vi "rosbridge.vi"() -> ()   [LabVIEW 2015]
uses:
  szablon odometry_filtered_local.ctl
  Gobal for ROS.vi
  Zmienne/longitude.vi
  Zmienne/latitude.vi
  szablon odometry_filtered_local.vi
  <vilib>/Intelligent Energy/WebSockets API/WebSockets/WebSockets.lvlib
  Zmienne globalne.lvlib
panel:
  out "x-y":u32
  out "value 2":T1
  in  "szablon odometry/filtered/local":T1
  in  "ROS data IMU":T2={"topic"="", "msg"={"header"={"seq"=63049, "stamp"={"secs"=0, "nsecs"=0}, "frame_id"="imu_link"}, "orientation"={"x"=0.0, "y"=0.0, "z"=0.0, "w"=0.0}, "orientation_covariance"=[], "angular_velocity"={"x"=0.0, "y"=0.0, "z"=0.0}, "angular_velocity_covariance"=[], "linear_acceleration"={"x"=0.0, "y"=0.0, "z"=0.0}, "linear_acceleration_covariance"=[]}, "op"=""}
  out "raw frame 2":string
  in  "STOP ROS READ 2":bool
  in  "ROS data read prędkości kół":T3
  out "error out 3":errorcluster
  in  "Topic string 2":string="{ \"op\": \"subscribe\", \"topic\" : \"/odometry/filtered/local\" }"
  in  "ROSB READ 2":bool
  in  "ROS data read 3":T4
  out "ROS data read 2":T5
  out "raw frame":string
  in  "STOP ROS READ":bool
  out "value":T6
  out "ROS data read":T7
  out "error out 2":errorcluster
  in  "Topic string":string="{ \"op\": \"subscribe\", \"topic\" : \"/fix\" }"
  in  "ROSB READ":bool
  # "Topic /fix na gpsa \ntopic rio/odom na prędkości\nIMU /data"
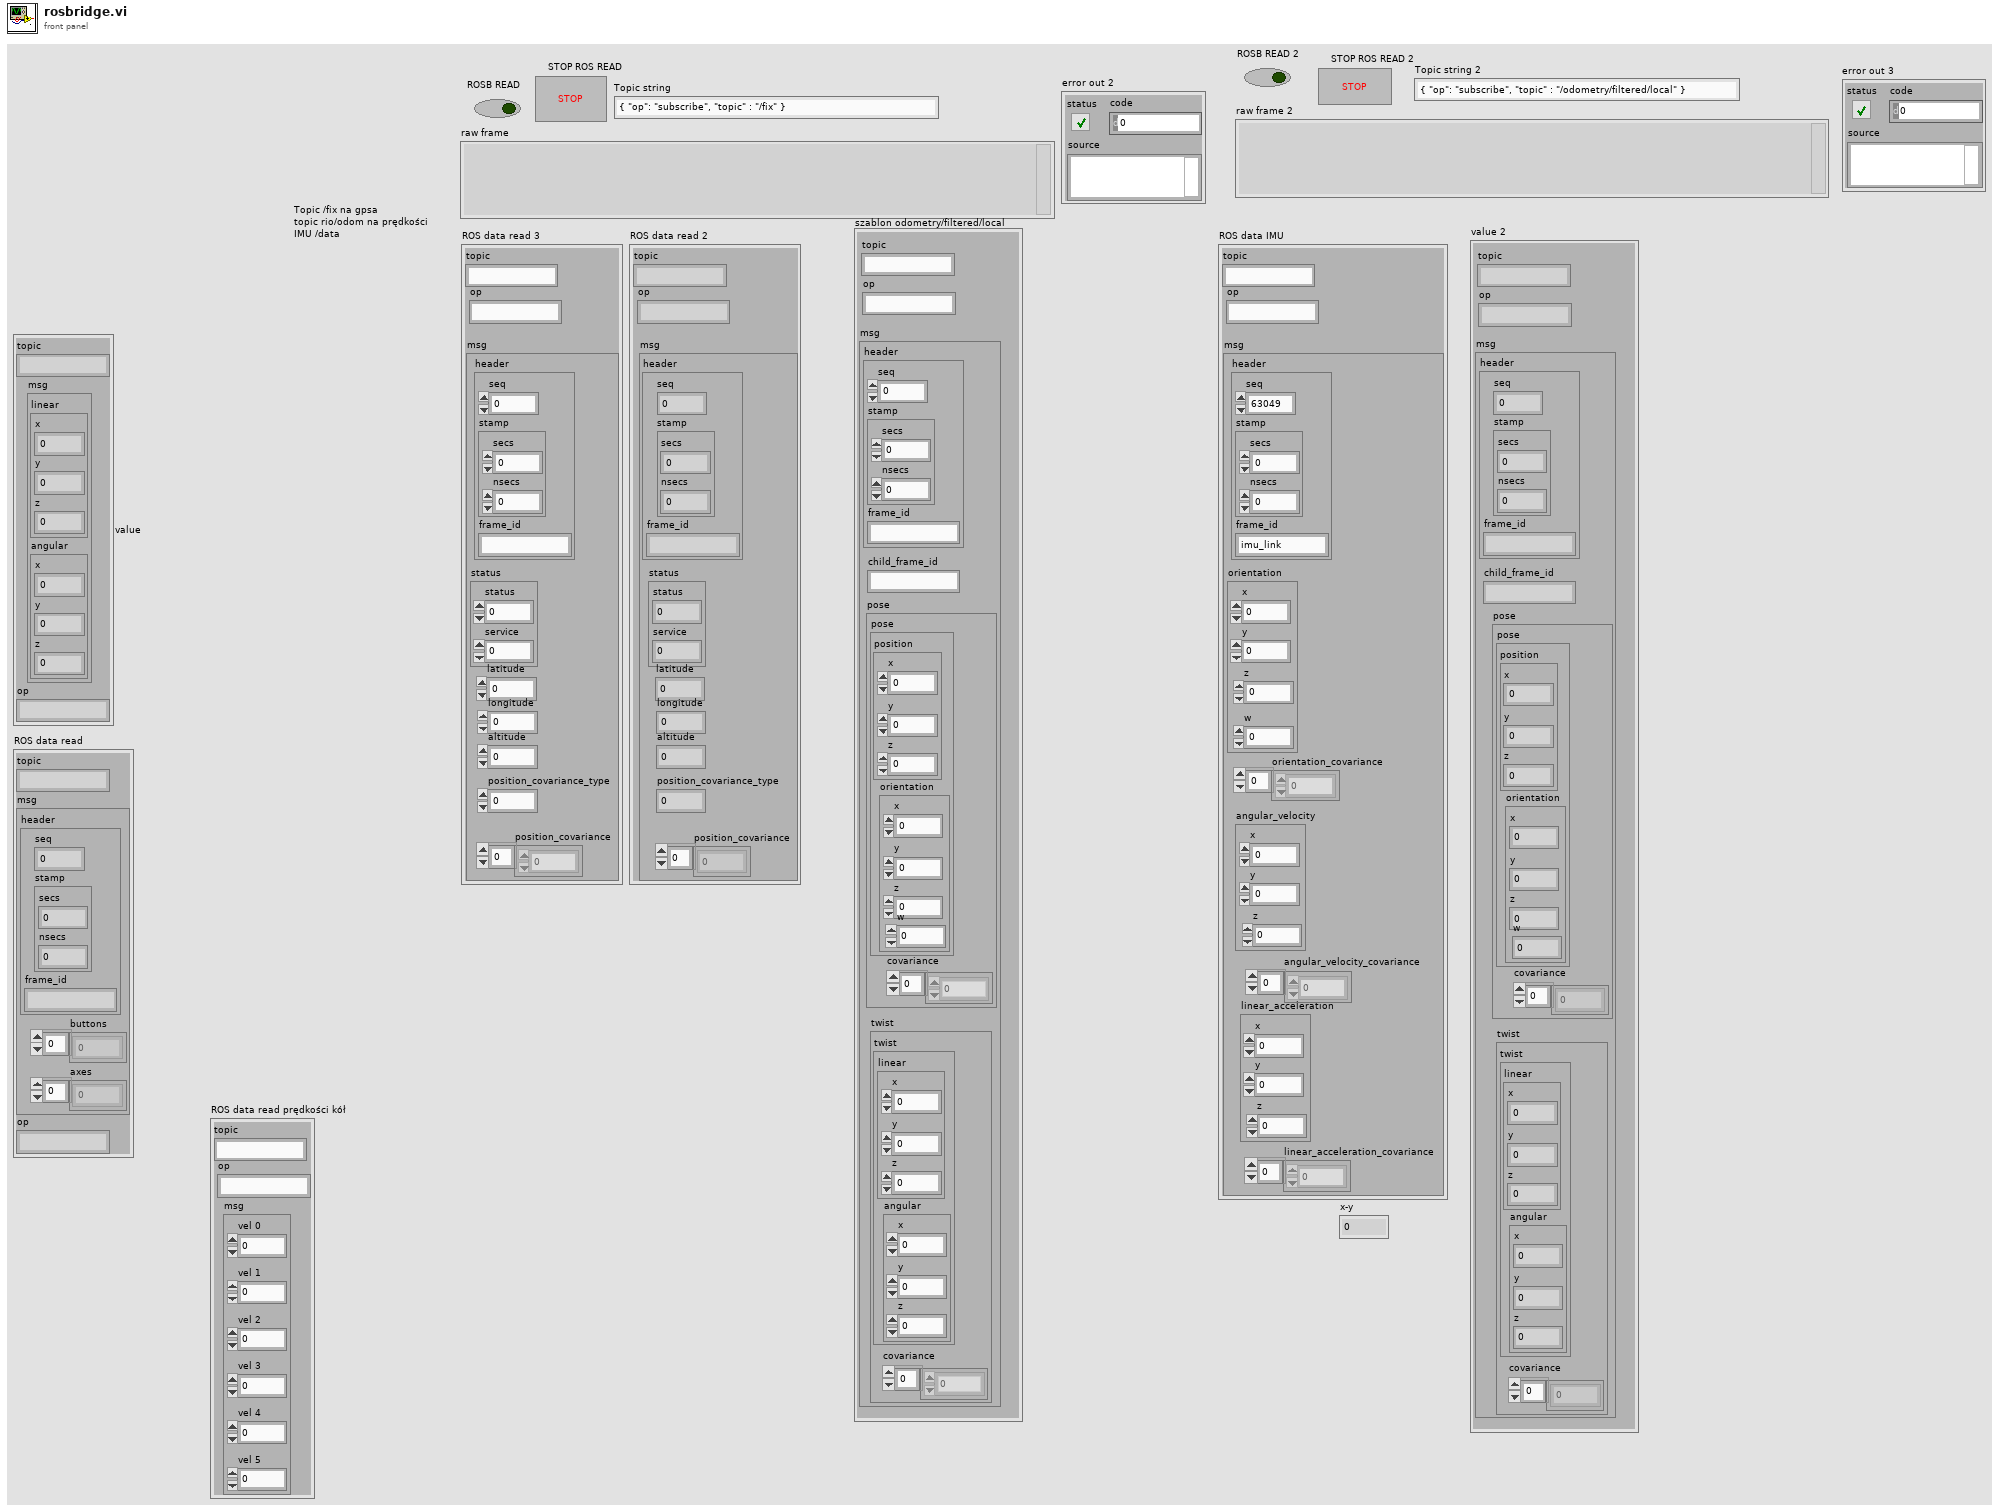
[diagram p1: front panel]
types:
  T1 = typedef "Biblioteka moduł map v3.lvlib/Zmienne globalne.lvlib/szablon odometry_filtered_local.ctl" = cluster{"topic":string, "msg":cluster{"header":cluster{"seq":u32, "stamp":cluster{"secs":u32, "nsecs":i32}, "frame_id":string}, "child_frame_id":string, "pose":cluster{"pose":cluster{"position":cluster{"y":dbl, "z":dbl, "x":dbl}, "orientation":cluster{"y":dbl, "z":dbl, "x":dbl, "w":dbl}}, "covariance":dbl[]}, "twist":cluster{"twist":cluster{"linear":cluster{"y":dbl, "z":dbl, "x":dbl}, "angular":cluster{"y":dbl, "z":dbl, "x":dbl}}, "covariance":dbl[]}}, "op":string}
  T2 = cluster{"topic":string, "msg":cluster{"header":cluster{"seq":u32, "stamp":cluster{"secs":u32, "nsecs":i32}, "frame_id":string}, "orientation":cluster{"x":dbl, "y":dbl, "z":dbl, "w":dbl}, "orientation_covariance":dbl[], "angular_velocity":cluster{"x":dbl, "y":dbl, "z":dbl}, "angular_velocity_covariance":dbl[], "linear_acceleration":cluster{"x":dbl, "y":dbl, "z":dbl}, "linear_acceleration_covariance":dbl[]}, "op":string}
  T3 = cluster{"topic":string, "msg":cluster{"vel 0":i64, "vel 1":i64, "vel 2":i64, "vel 3":i64, "vel 4":i64, "vel 5":i64}, "op":string}
  T4 = cluster{"topic":string, "msg":cluster{"header":cluster{"seq":u32, "stamp":cluster{"secs":u32, "nsecs":i32}, "frame_id":string}, "status":cluster{"status":u32, "service":i32}, "position_covariance":dbl[], "latitude":dbl, "longitude":dbl, "altitude":i32, "position_covariance_type":dbl}, "op":string}
  T5 = cluster{"topic":string, "msg":cluster{"header":cluster{"seq":u32, "stamp":cluster{"secs":u32, "nsecs":i32}, "frame_id":string}, "status":cluster{"status":u32, "service":i32}, "position_covariance":sgl[], "latitude":dbl, "longitude":dbl, "altitude":i32, "position_covariance_type":i32}, "op":string}
  T6 = cluster{"topic":string, "msg":cluster{"linear":cluster{"x":dbl, "y":dbl, "z":dbl}, "angular":cluster{"x":dbl, "y":dbl, "z":dbl}}, "op":string}
  T7 = cluster{"topic":string, "msg":cluster{"header":cluster{"seq":u32, "stamp":cluster{"secs":u32, "nsecs":i32}, "frame_id":string}, "buttons":i32[], "axes":sgl[]}, "op":string}
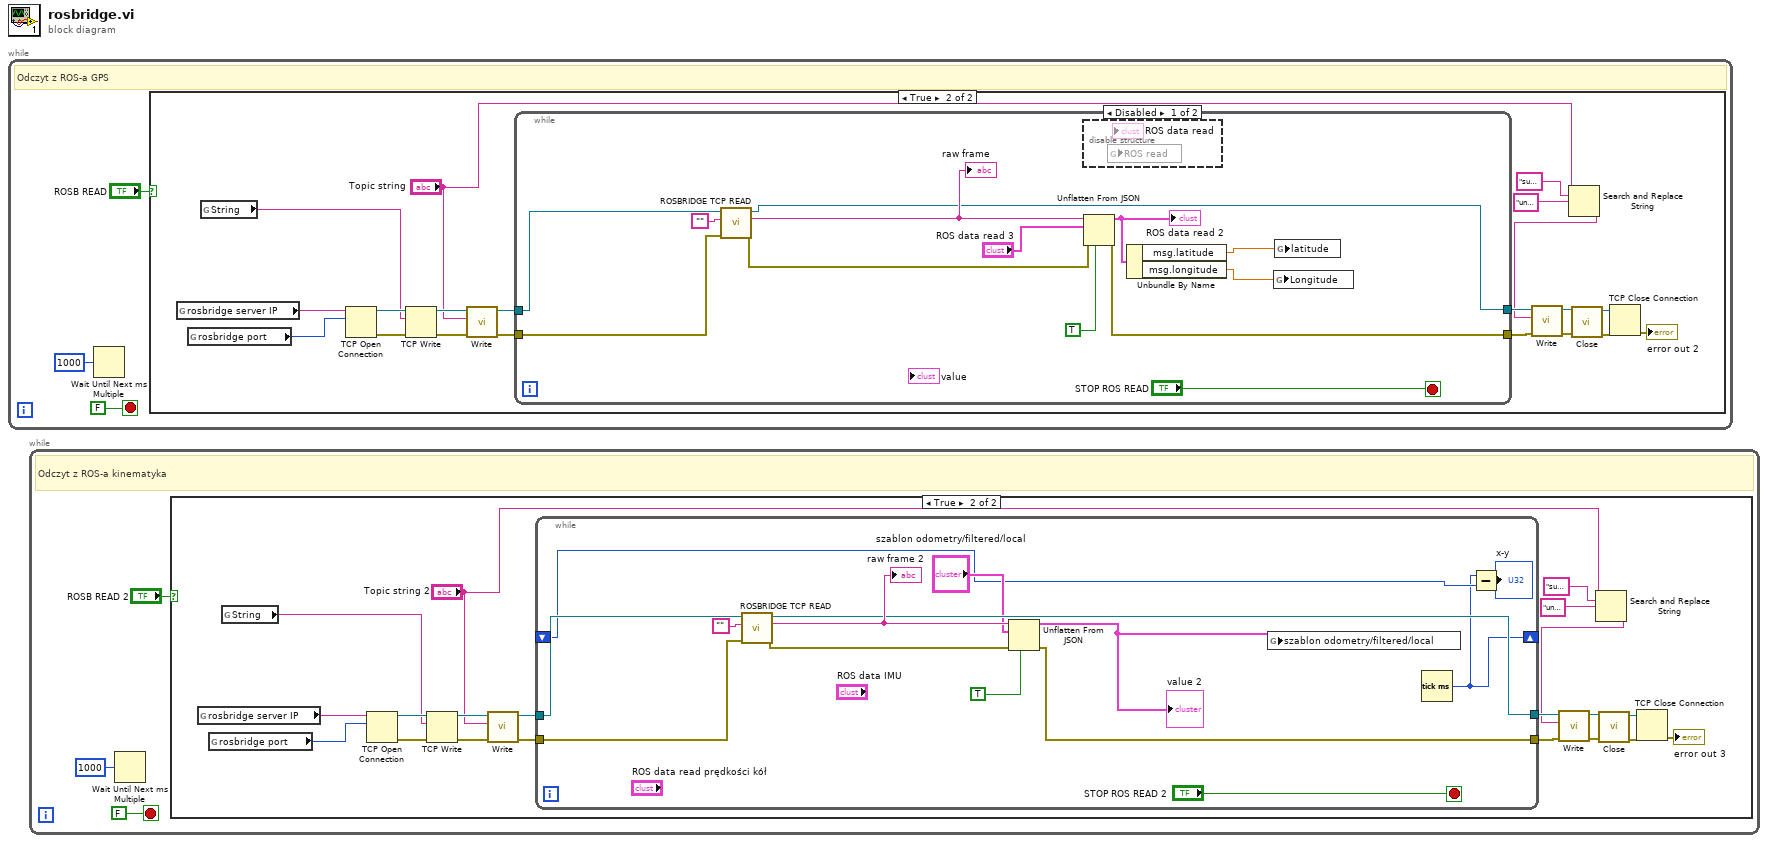
[diagram p0: block diagram]
diagram:
  n1 = while {
    stop <- FALSE stop-if-true
    # "Odczyt z ROS-a GPS"
    n2 = Wait Until Next ms Multiple(millisecond multiple=u32 1000 ("milliseconds to wait")) -> ()  [unwired: 1 out]
    n3 = case shown="True" "ROSB READ" {
      frame False {
      }
      frame True {
        n4 = global read "Gobal for ROS.vi" "rosbridge server IP"() -> (w13:string)
        n5 = global read "Gobal for ROS.vi" "rosbridge port"() -> (w12:u16)
        n6 = global read "Gobal for ROS.vi" "String"() -> (w14:string)
        n7 = TCP Open Connection(address=w13, remote port or service name=w12) -> (connection ID=w23:refnum<k5>, error out=w22:errorcluster)  [unwired: 3 in]
        n8 = TCP Write(connection ID=w23, data in=w14, error in (no error)=w22) -> (connection ID out=w19:refnum<k5>, error out=w18:errorcluster)  [unwired: 1 in, 1 out]
        n9 = call <vilib>:"Write.vi"("error in (no error)"=w18, "Data"="Topic string", "WebSocket Connection in"=w19) -> ("error out"=w16:errorcluster, "WebSocket Connection out"=w17:refnum<k5>)  [unwired: 7 in]
        n10 = while {
          tunnel: [w29] -> w9
          tunnel: [w36] -> w8
          tunnel: w17 -> [w31]
          tunnel: w16 -> [w30]
          stop <- "STOP ROS READ" stop-if-true
          n11 = call "ROSBRIDGE TCP READ.vi"("error in (no error)"=w30, "String in"="", "TCP Network Connection in"=w31) -> ("error out"=w28:errorcluster, "String out"=w32:string, "TCP Network Connection out"=w29:refnum<k5>)  [unwired: 6 in]
          "raw frame" <- w32
          n12 = disable-structure shown="Disabled" {
            frame Disabled {
              n13 = global read "Gobal for ROS.vi" "ROS read"() -> ()  [unwired: 1 in]
            }
            frame Enabled {
            }
          }
          n14 = Unflatten From JSON(JSON string=w32, type and defaults="ROS data read 3", default null elements? (F)=TRUE, error in (no error)=w28) -> (value=w26:T4, error out=w36:errorcluster)  [unwired: 3 in]
          "ROS data read 2" <- w26
          n15 = Unbundle By Name(w26) -> ("msg.latitude"=w25:dbl, "msg.longitude"=w24:dbl)
          n16 = global write "longitude.vi" "Longitude"(w24) -> ()
          n17 = global write "latitude.vi" "latitude"(w25) -> ()
        }
        n18 = Search and Replace String(input string="Topic string", search string="subscribe", replace string="unsubscribe" ("search string")) -> (result string=w7:string)  [unwired: 5 in, 3 out]
        n19 = call <vilib>:"Write.vi"("error in (no error)"=w8, "Data"=w7, "WebSocket Connection in"=w9) -> ("error out"=w10:errorcluster, "WebSocket Connection out"=w11:refnum<k5>)  [unwired: 7 in]
        n20 = call <vilib>:"Close.vi"("error in (no error)"=w10, "WebSocket Connection in"=w11) -> ("error out"=w20:errorcluster, "WebSocket Connection in"=w21:refnum<k5>)  [unwired: 8 in]
        n21 = TCP Close Connection(connection ID=w21, error in (no error)=w20) -> (error out=→"error out 2":errorcluster)  [unwired: 1 in, 1 out]
      }
    }
  }
  n22 = while {
    stop <- FALSE stop-if-true
    # "Odczyt z ROS-a kinematyka"
    n23 = Wait Until Next ms Multiple(millisecond multiple=u32 1000 ("milliseconds to wait")) -> ()  [unwired: 1 out]
    n24 = case shown="True" "ROSB READ 2" {
      frame False {
      }
      frame True {
        n25 = global read "Gobal for ROS.vi" "rosbridge server IP"() -> (w49:string)
        n26 = global read "Gobal for ROS.vi" "rosbridge port"() -> (w48:u16)
        n27 = global read "Gobal for ROS.vi" "String"() -> (w50:string)
        n28 = TCP Open Connection(address=w49, remote port or service name=w48) -> (connection ID=w59:refnum<k5>, error out=w58:errorcluster)  [unwired: 3 in]
        n29 = TCP Write(connection ID=w59, data in=w50, error in (no error)=w58) -> (connection ID out=w55:refnum<k5>, error out=w54:errorcluster)  [unwired: 1 in, 1 out]
        n30 = call <vilib>:"Write.vi"("error in (no error)"=w54, "Data"="Topic string 2", "WebSocket Connection in"=w55) -> ("error out"=w52:errorcluster, "WebSocket Connection out"=w53:refnum<k5>)  [unwired: 7 in]
        n31 = while {
          tunnel: [w66] -> w45
          tunnel: [w73] -> w44
          tunnel: w53 -> [w68]
          tunnel: w52 -> [w67]
          shift-right: [w60] -> _
          shift-left: _ -> [w61]
          stop <- "STOP ROS READ 2" stop-if-true
          n32 = call "ROSBRIDGE TCP READ.vi"("error in (no error)"=w67, "String in"="", "TCP Network Connection in"=w68) -> ("error out"=w65:errorcluster, "String out"=w69:string, "TCP Network Connection out"=w66:refnum<k5>)  [unwired: 6 in]
          "raw frame 2" <- w69
          n33 = Unflatten From JSON(JSON string=w69, type and defaults="szablon odometry/filtered/local", default null elements? (F)=TRUE, error in (no error)=w65) -> (value=w64:T1, error out=w73:errorcluster)  [unwired: 3 in]
          "value 2" <- w64
          n34 = global write "szablon odometry_filtered_local.vi" "szablon odometry/filtered/local"(w64) -> ()
          n35 = Tick Count (ms)() -> (millisecond timer value=w60:u32)
          n36 = Subtract(x=w60, y=w61) -> (x-y=→"x-y":u32)
        }
        n37 = Search and Replace String(input string="Topic string 2", search string="subscribe", replace string="unsubscribe" ("search string")) -> (result string=w43:string)  [unwired: 5 in, 3 out]
        n38 = call <vilib>:"Write.vi"("error in (no error)"=w44, "Data"=w43, "WebSocket Connection in"=w45) -> ("error out"=w46:errorcluster, "WebSocket Connection out"=w47:refnum<k5>)  [unwired: 7 in]
        n39 = call <vilib>:"Close.vi"("error in (no error)"=w46, "WebSocket Connection in"=w47) -> ("error out"=w56:errorcluster, "WebSocket Connection in"=w57:refnum<k5>)  [unwired: 8 in]
        n40 = TCP Close Connection(connection ID=w57, error in (no error)=w56) -> (error out=→"error out 3":errorcluster)  [unwired: 1 in, 1 out]
      }
    }
  }
